vi "Parse Value.vi"(11 "Value":string) -> (2 "Value (Comment Removed)":string, 3 "Value (Quotes Removed)":string)   [LabVIEW 2022 SP3, in "LabVIEW-Config.lvlib"]
uses:
  LabVIEW-Config.lvlib
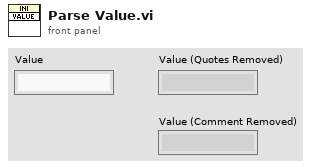
[diagram p1: front panel]
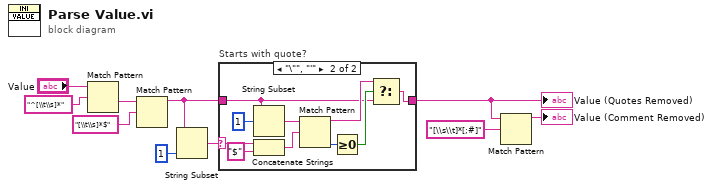
[diagram p0: block diagram]
diagram:
  n1 = Match Pattern(string="Value", regular expression="^[\\t\\s]*") -> (after substring=w5:string)  [unwired: 1 in, 3 out]
  n2 = Match Pattern(string=w5, regular expression="[\\t\\s]*$") -> (before substring=w4:string)  [unwired: 1 in, 3 out]
  n3 = String Subset(string=w4, length (rest)=1 ("length (rest)")) -> (substring=w9:string)  [unwired: 1 in]
  n4 = case "Starts with quote?" shown="\"\\\"\", \"'\"" w9 {
    selector: w9 -> [_ w14]
    tunnel: [w11 w15] -> w3
    tunnel: w4 -> [w11 w16]
    frame Default {
    }
    frame "\"", "'" {
      n5 = String Subset(string=w16, offset (0)=1 ("length (rest)")) -> (substring=w20:string)  [unwired: 1 in]
      n6 = Concatenate Strings(w14, "$" ("string")) -> (w12:string)
      n7 = Match Pattern(string=w20, regular expression=w12) -> (before substring=w17:string, offset past match=w19:i32)  [unwired: 1 in, 2 out]
      n8 = Greater Or Equal To 0?(x=w19) -> (x >= 0?=w18:bool)
      n9 = Select(t=w17, s=w18, f=w16) -> (s? t:f=w15:string)
    }
  }
  "Value (Quotes Removed)" <- w3
  n10 = Match Pattern(string=w3, regular expression="[\\s\\t]*[;#]") -> (before substring=→"Value (Comment Removed)":string)  [unwired: 1 in, 3 out]
